vi "NewEntry_DB.vi"(8 "error in (no error)":errorcluster, 11 "LotData in":refnum<class "LotData.lvclass">) -> (0 "error out":errorcluster, 2 "NewWaferEntry":string, 3 "LotData out":refnum<class "LotData.lvclass">)   [LabVIEW 2012, in "LotData.lvclass"]
uses:
  LotData.lvclass
  LotData.lvclass/LotData.ctl
  <vilib>/addons/database/Auxilliary.llb/DB Tools Parameter Info.ctl
  <vilib>/addons/database/Auxilliary.llb/DB Tools DataTypes.ctl
  <vilib>/addons/database/Auxilliary.llb/DB Tools Parameter Dir.ctl
  <vilib>/addons/database/Connection.llb/DB Tools Open Connec (Path).vi
  <vilib>/addons/database/Command.llb/Cmd Set Parameter Value (C).vi
  <vilib>/addons/database/Command.llb/Cmd Execute.vi
  <vilib>/addons/database/Recordset.llb/Rec Destroy - Command.vi
  <vilib>/addons/database/Command.llb/Cmd Delete.vi
  <vilib>/addons/database/NI_Database_API.lvlib
panel:
  out "Pocket":string
  out "Run Number":string
  out "System":string
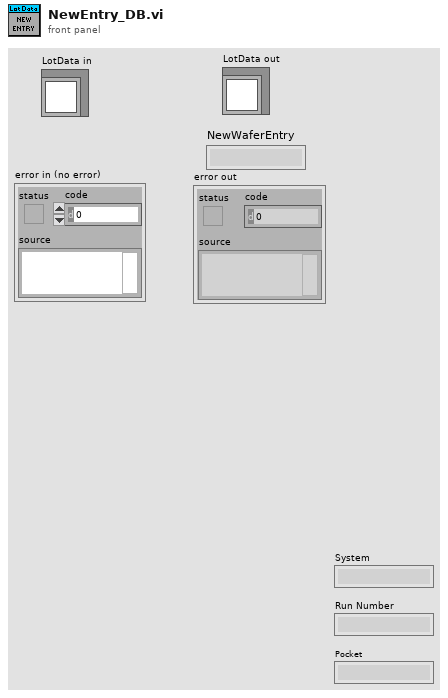
[diagram p1: front panel]
types:
  T1 = typedef "NI_Database_API.lvlib/DB Tools Parameter Info.ctl" = cluster{"parameter name":string, "type":T2, "direction":T3, "value":variant}
  T2 = typedef "NI_Database_API.lvlib/DB Tools DataTypes.ctl" = enum16{"String", "Long (I32)", "Single (SGL)", "Double (DBL)", "Date/Time", "Binary"}
  T3 = typedef "NI_Database_API.lvlib/DB Tools Parameter Dir.ctl" = enum32{"Input", "Output", "Input/Output", "Return Value"}
  T4 = typedef "NI_Database_API.lvlib/Conn ObjectReference.ctl" = refnum<k1>
  T5 = typedef "NI_Database_API.lvlib/Cmd ObjectReference.ctl" = refnum<k1>
  T6 = typedef "NI_Database_API.lvlib/Cmd-Rec Object Reference.ctl" = refnum<k1>
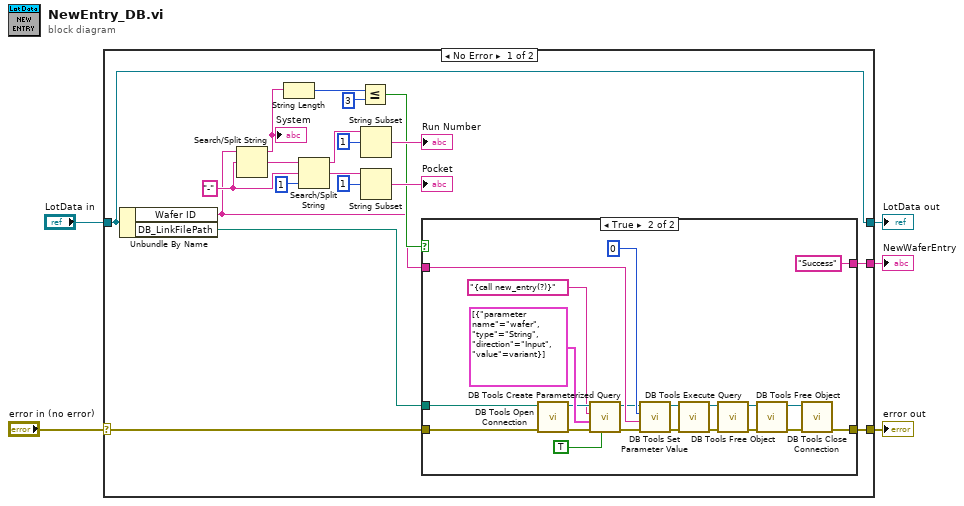
[diagram p0: block diagram]
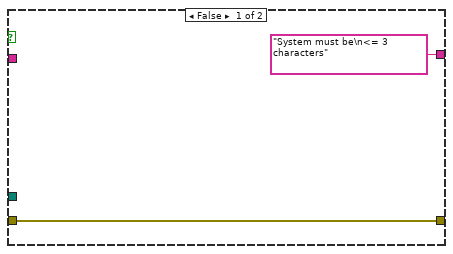
[diagram p2: hidden frame]
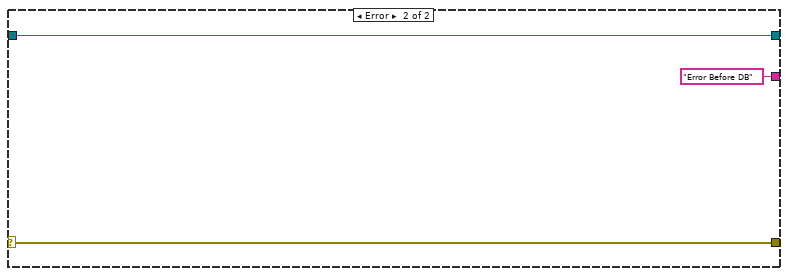
[diagram p3: hidden frame]
diagram:
  n1 = case shown="No Error" "error in (no error)" {
    selector: "error in (no error)" -> [w7 w50]
    tunnel: [w9 w50] -> w2
    tunnel: [w24 w49] -> w3
    tunnel: "LotData in" -> [w24 w49]
    tunnel: [w8 "Error Before DB" ("NewWaferEntry")] -> w1
    frame No Error {
      w22 = "-" ("search string/char (-)")
      n2 = Unbundle By Name(w24) -> ("Wafer ID"=w10:string, "DB_LinkFilePath"=w6:path)
      n3 = Search/Split String(string=w10, search string/char (-)=w22) -> (substring before match=w14:string, match + rest of string=w23:string)  [unwired: 1 in, 1 out]
      "System" <- w14
      n4 = String Length(string=w14) -> (length=w13:i32)
      n5 = Search/Split String(string=w23, search string/char (-)=w22, offset (0)=1) -> (substring before match=w17:string, match + rest of string=w20:string)  [unwired: 1 out]
      n6 = Less Or Equal?(x=w13, y=3) -> (x <= y?=w11:bool)
      n7 = String Subset(string=w17, offset (0)=1) -> (substring=→"Run Number":string)  [unwired: 1 in]
      n8 = String Subset(string=w20, offset (0)=1) -> (substring=→"Pocket":string)  [unwired: 1 in]
      n9 = case shown="True" w11 {
        tunnel: w10 -> [_ w41]
        tunnel: [w26 w37] -> w9
        tunnel: w7 -> [w26 w30]
        tunnel: ["System must be\n<= 3 characters" "Success"] -> w8
        tunnel: w6 -> [_ w27]
        frame False {
        }
        frame True {
          n10 = call-poly <vilib>:"DB Tools Open Connection.vi"("error in (no error)"=w30, "connection information"=w27) -> ("error out"=w44:errorcluster, "connection reference"=w45:T4)  [unwired: 6 in]
          n11 = call <vilib>:"DB Tools Create Parameterized Query.vi"("stored procedure? (F)"=TRUE, "error in (no error)"=w44, "parameters"=T1[] [{"parameter name"="wafer", "type"=enum."String", "direction"=enum."Input", "value"=variant}], "SQL query"="{call new_entry(?)}", "connection reference"=w45) -> ("error out"=w40:errorcluster, "command reference"=w39:T5)  [unwired: 2 in, 1 out]
          n12 = call-poly <vilib>:"DB Tools Set Parameter Value.vi"("error in (no error)"=w40, "value"=w41, "parameter index"=0, "command reference"=w39) -> ("error out"=w34:errorcluster, "command reference out"=w35:T5)  [unwired: 4 in]
          n13 = call-poly <vilib>:"DB Tools Execute Query.vi"("error in (no error)"=w34, "command reference"=w35) -> ("error out"=w33:errorcluster, "command-recordset reference"=w36:T6)  [unwired: 6 in]
          n14 = call-poly <vilib>:"DB Tools Free Object.vi"("error in (no error)"=w33, "command-recordset reference"=w36) -> ("error out"=w38:errorcluster, "command reference"=w28:T5)  [unwired: 8 in]
          n15 = call-poly <vilib>:"DB Tools Free Object.vi"("error in (no error)"=w38, "command reference"=w28) -> ("error out"=w31:errorcluster, "connection reference"=w32:T4)  [unwired: 8 in]
          n16 = call <vilib>:"DB Tools Close Connection.vi"("error in (no error)"=w31, "connection reference"=w32) -> ("error out"=w37:errorcluster)  [unwired: 5 in]
        }
      }
    }
    frame Error {
    }
  }
  "error out" <- w2
  "LotData out" <- w3
  "NewWaferEntry" <- w1
